vi "Power Peak Calibration Inputs.vi"(1 "Input":dbl format="%#_13g", 2 "Calibration Input FGV Selector":T1, 3 "Verb":T2) -> (0 "Output":dbl format="%#_13g")   [LabVIEW 2013]
uses:
  Action.ctl
  Power Peak Calibration Input FGV Selector.ctl
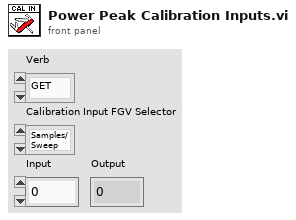
[diagram p1: front panel]
types:
  T1 = typedef "Power Peak Calibration Input FGV Selector.ctl" = enum16{"Samples/Sweep", "Num Sweeps", "Sample Rate"}
  T2 = typedef "Action.ctl" = enum16{"GET", "PUT", "DELETE"}
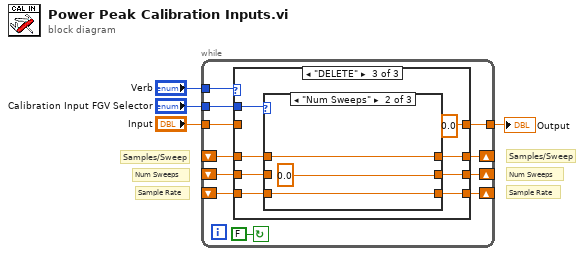
[diagram p0: block diagram]
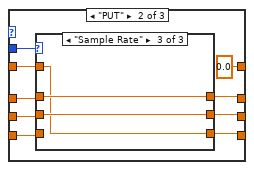
[diagram p5: hidden frame]
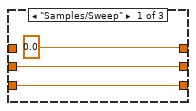
[diagram p8: hidden frame]
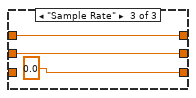
[diagram p9: hidden frame]
diagram:
  # "Num Sweeps"
  # "Sample Rate"
  # "Samples/Sweep"
  # "Num Sweeps"
  # "Sample Rate"
  # "Samples/Sweep"
  n1 = while {
    shift-right: [w7] -> _
    shift-left: _ -> [w10]
    shift-right: [w6] -> _
    shift-left: _ -> [w9]
    shift-right: [w5] -> _
    shift-left: _ -> [w8]
    tunnel: "Input" -> [w12]
    tunnel: "Calibration Input FGV Selector" -> [w13]
    tunnel: "Verb" -> [w14]
    tunnel: [w11] -> w1
    stop <- FALSE continue-if-true
    n2 = case shown="\"DELETE\"" w14 {
      tunnel: w13 -> [w23 w41 w58]
      tunnel: w12 -> [_ w33 _]
      tunnel: [w16 0.0 0.0] -> w11
      tunnel: w10 -> [w21 w40 w57]
      tunnel: w9 -> [w19 w39 w56]
      tunnel: w8 -> [w17 w38 w55]
      tunnel: [w22 w37 w53] -> w7
      tunnel: [w20 w36 w54] -> w6
      tunnel: [w18 w35 w51] -> w5
      frame "GET", Default {
        n3 = case shown="\"Samples/Sweep\"" w23 {
          tunnel: [w24 w29 w32] -> w22
          tunnel: w21 -> [w24 w29 w32]
          tunnel: [w26 w27 w31] -> w20
          tunnel: w19 -> [w26 w27 w31]
          tunnel: [w25 w28 w30] -> w18
          tunnel: w17 -> [w25 w28 w30]
          tunnel: [w24 w27 w30] -> w16
          frame "Samples/Sweep" {
          }
          frame "Num Sweeps" {
          }
          frame "Sample Rate" {
          }
        }
      }
      frame "PUT" {
        n4 = case shown="\"Sample Rate\"" w41 {
          tunnel: [w42 w47 w50] -> w37
          tunnel: w40 -> [_ w47 w50]
          tunnel: [w44 w45 w49] -> w36
          tunnel: w39 -> [w44 _ w49]
          tunnel: [w43 w46 w48] -> w35
          tunnel: w38 -> [w43 w46 _]
          tunnel: w33 -> [w42 w45 w48]
          frame "Samples/Sweep" {
          }
          frame "Num Sweeps" {
          }
          frame "Sample Rate" {
          }
        }
      }
      frame "DELETE" {
        n5 = case shown="\"Num Sweeps\"" w58 {
          tunnel: w57 -> [_ w64 w66]
          tunnel: w56 -> [w61 _ w67]
          tunnel: w55 -> [w60 w63 _]
          tunnel: [w61 0.0 w67] -> w54
          tunnel: [0.0 w64 w66] -> w53
          tunnel: [w60 w63 0.0] -> w51
          frame "Samples/Sweep" {
          }
          frame "Num Sweeps" {
          }
          frame "Sample Rate" {
          }
        }
      }
    }
  }
  "Output" <- w1
